vi "Async Read&Write.vi"(1 "Minor Frame Freq":u16 caption="Minor Frame Time", 4 "Frame Info Array":T1[](array[typedef]), 5 "Port":string, 6 "Stop Notification":refnum<notifier>, 7 "Main Engine Response Q":refnum<queue>, 8 "error in":errorcluster, 9 "Interupt Q":refnum<queue>, 10 "TCP Engine Response Q":refnum<queue>, 11 "Data Cluster":T3={"Array"=[], "Boolean"=FALSE, "Varient Data"=variant(string ""), "Stop Notification"=refnum, "Start Notification"=refnum, "Command Q"=refnum, "Main Engine Response Q"=refnum, "TCP Engine Response Q"=refnum, "Engine Name"="", "Log File Refnum"=refnum, "Async serial Configuration Cluster"={"Port"="", "Minor Frame Freq"=0, "Minor Frame Count"=0, "Frame Info"=[], "Sensor Type"=0, "OIM Address"=0}, "VISA resource name"="", "Y"=[], "Rate"=0, "Dynamic Data?"=FALSE, "DyData Not Received"=FALSE, "Interupt Q"=refnum, "Modbus"=refnum} {"Async serial Configuration Cluster"."Minor Frame Count" min=5 max=8 step=1}) -> (0 "error out":errorcluster, 2 "Total # Send":i32, 3 "Device Stop":bool)   [LabVIEW 2024]
doc: "All Rights Reserved © 2017 SyncSols"
uses:
  TCP Engine/Controls/TCP Engine Serial Interupt Cluster.ctl
  Controls/Async Frame Info Cluster.ctl
  Controls/Async Message Info Cluster.ctl
  Controls/Async Serial State Machine Data Cluster.ctl
  <vilib>/Modbus/master/Modbus Master.lvclass
  Controls/Async Serial Command Q Cluster.ctl
  Controls/Async Serial Configuration Cluster.ctl
  Main Engine/Controls/Main Engine JSON Command State.ctl
  Controls/Async Sensor Type.ctl
  <vilib>/Platform/TimedLoop/XDataNode/timing_clust.ctl
  <vilib>/Platform/TimedLoop/XDataNode/nitl_modes.ctl
  <vilib>/Platform/TimedLoop/XDataNode/wakeup.ctl
  1c283609-df89-4253-93f7-a40e07c9ee0e.vi
  <vilib>/Platform/TimedLoop/XDataNode/XDataNode.xnode
  <vilib>/Platform/TimedLoop/XDataNode/XDNodeRunTimeDep.lvlib
  TCP Engine/TCP Engine.lvlib
panel:
  in  "Frame Info":T1[](array[typedef])=[{"Frame ID"=1, "Message Info"=[{"Message"=[0, 0, 0, 0, 0, 0], "Message Name"="Camera cmd 1"}, {"Message"=[0, 0, 0, 0, 0, 0], "Message Name"="Camera cmd 2"}]}]
  out "Stop":bool=TRUE
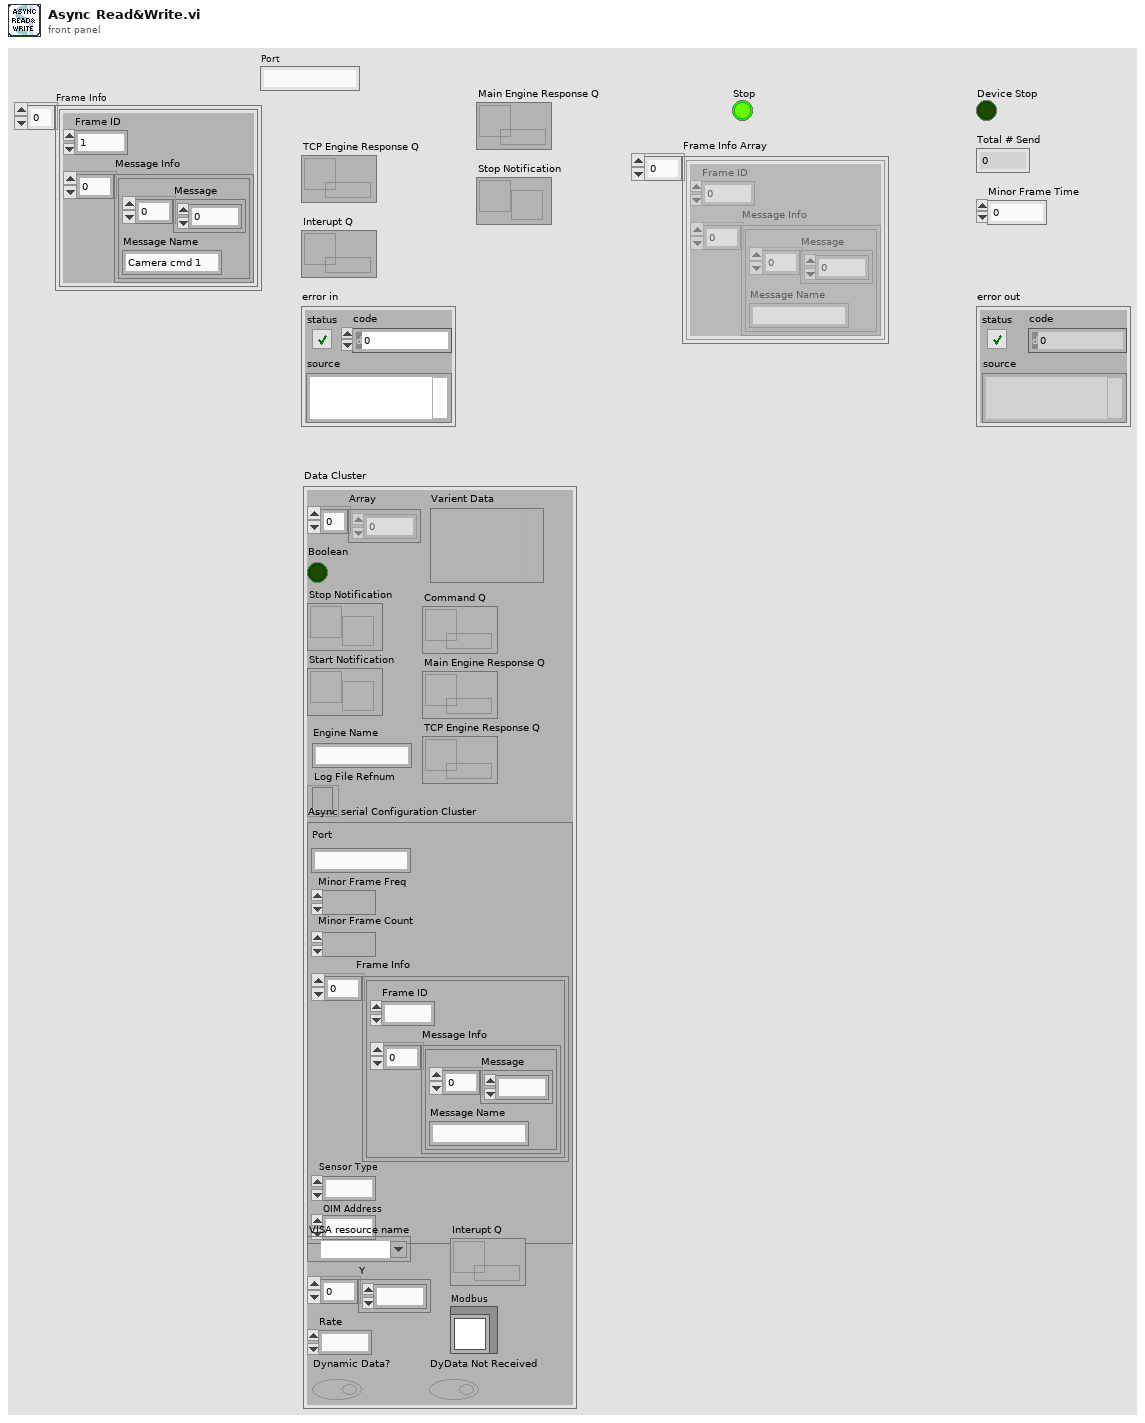
[diagram p1: front panel]
types:
  T1 = typedef "Async Frame Info Cluster.ctl" = cluster{"Frame ID":u16, "Message Info":T2[]}
  T2 = typedef "Async Message Info Cluster.ctl" = cluster{"Message":u8[], "Message Name":string}
  T3 = typedef "Async Serial State Machine Data Cluster.ctl" = cluster{"Array":dbl[], "Boolean":bool, "Varient Data":variant, "Stop Notification":refnum<notifier>, "Start Notification":refnum<notifier>, "Command Q":refnum<queue>, "Main Engine Response Q":refnum<queue>, "TCP Engine Response Q":refnum<queue>, "Engine Name":string, "Log File Refnum":refnum<file>, "Async serial Configuration Cluster":T4, "VISA resource name":refnum<visa-resource-name>, "Y":dbl[], "Rate":i32, "Dynamic Data?":bool, "DyData Not Received":bool, "Interupt Q":refnum<queue>, "Modbus":refnum<class "Modbus Master.lvclass">}
  T4 = typedef "Async Serial Configuration Cluster.ctl" = cluster{"Port":string, "Minor Frame Freq":u16, "Minor Frame Count":u16, "Frame Info":T1[], "Sensor Type":u16, "OIM Address":u16}
  T5 = typedef "Async Sensor Type.ctl" = enum16{"Camera", "INS", "Pri BMS", "Aux BMS", "Depth Sensor", "Altimeter", "OIM", "Thruster", "Acoustic Modem", "LED"}
  T6 = cluster{"Command":string, "SubCmd":string, "Data":cluster{"Port":string, "Length":u16, "Data":u8[], "Time":string}}
  T7 = typedef "XDNodeRunTimeDep.lvlib/timing_clust.ctl" = cluster{"Expected End [f-1]":u64, "Actual End [f-1]":u64, "Finished Late? [f-1]":bool, "Expected End [i-1]":u64, "Actual End [i-1]":u64, "Finished Late? [i-1]":bool, "Expected Start [i]":u64, "Actual Start [i]":u64, "Expected Start [f]":u64, "Actual Start [f]":u64, "Source Name":string, "Structure Name":string, "Period":i64, "Deadline":i64, "Offset":i64, "Start":i64, "Priority":i32, "Timeout":i32, "Mode":T8, "Wakeup Reason":T9, "Error":errorcluster, "Source Type":string, "Secondary Source Type":string, "Global End Time":u64, "Global Start Time":u64, "Frame Duration":u64, "Iteration Duration":u64, "Assigned CPU":i32, "I/O Scan Engine Mode":u32}
  T8 = typedef "XDNodeRunTimeDep.lvlib/nitl_modes.ctl" = enum32{"No Change", "Process missed periods, maintain original phase", "Discard missed periods, maintain original phase", "Process missed periods, ignore original phase", "Discard missed periods, ignore original phase"}
  T9 = typedef "XDNodeRunTimeDep.lvlib/wakeup.ctl" = enum32{"Normal", "Aborted", "Asynchronous wakeup", "Timing source error", "Timed loop error", "Timeout"}
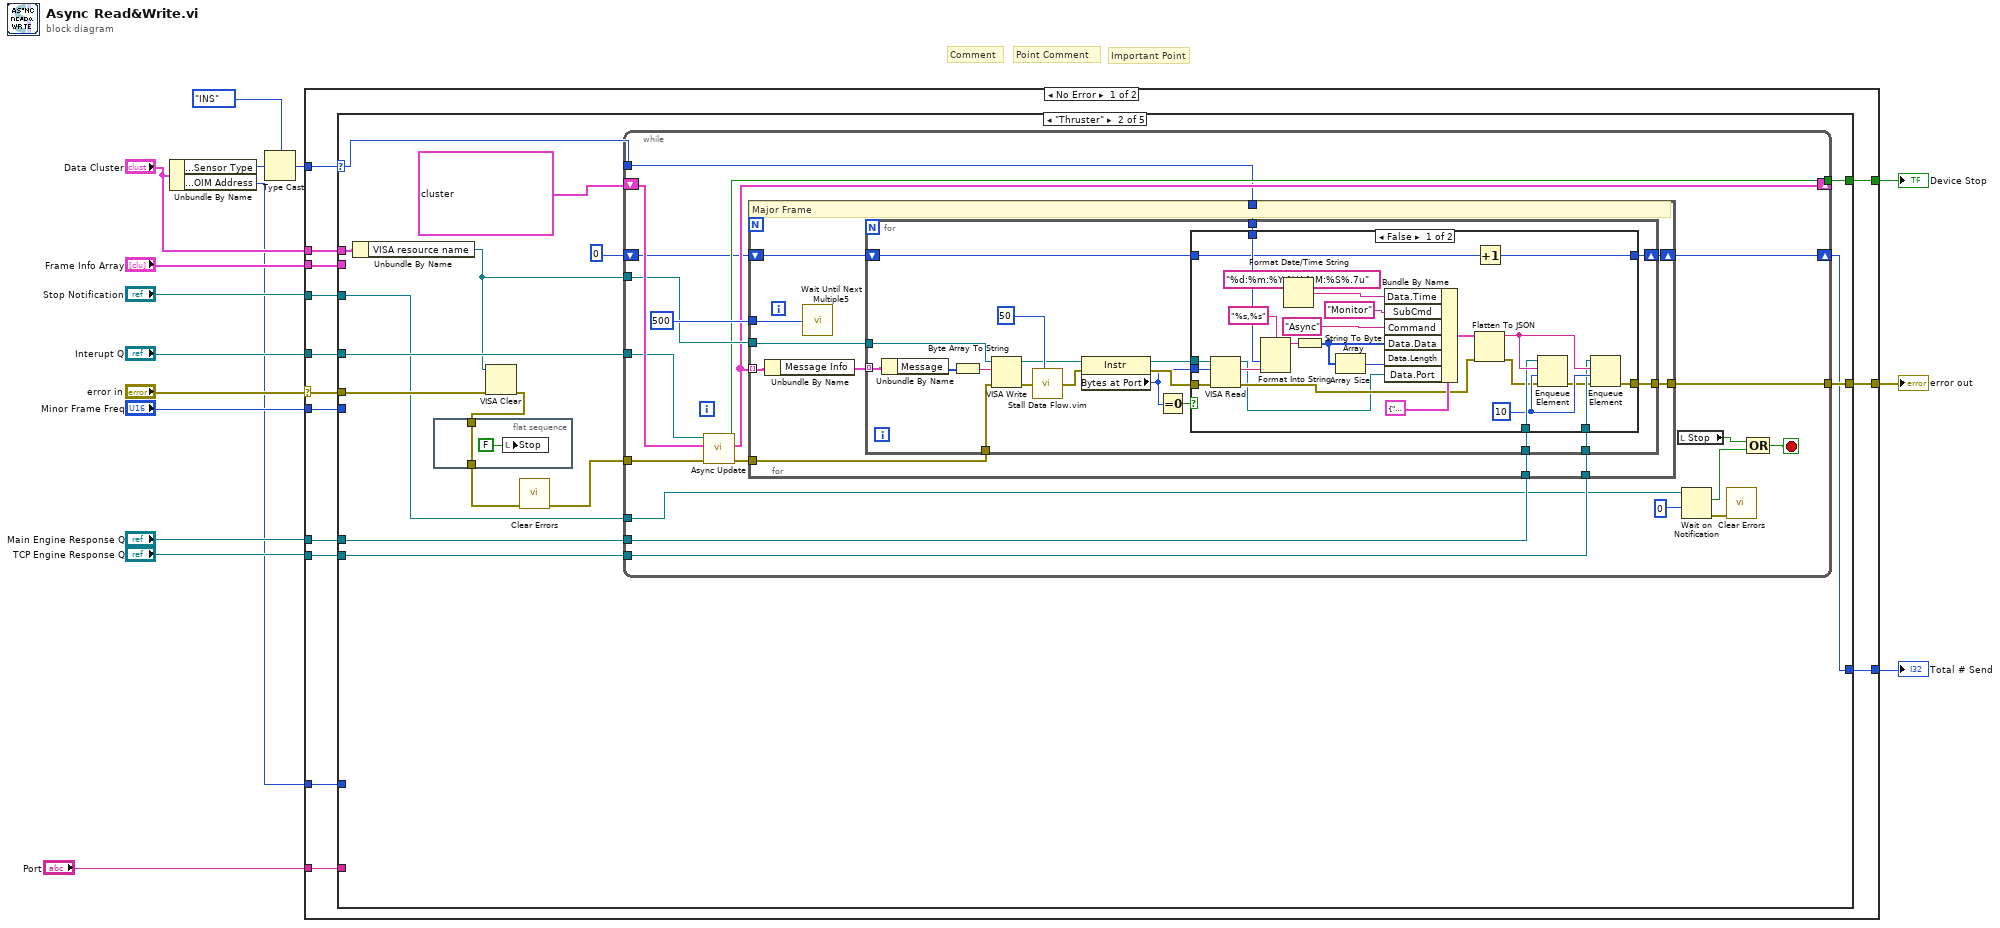
[diagram p0: block diagram]
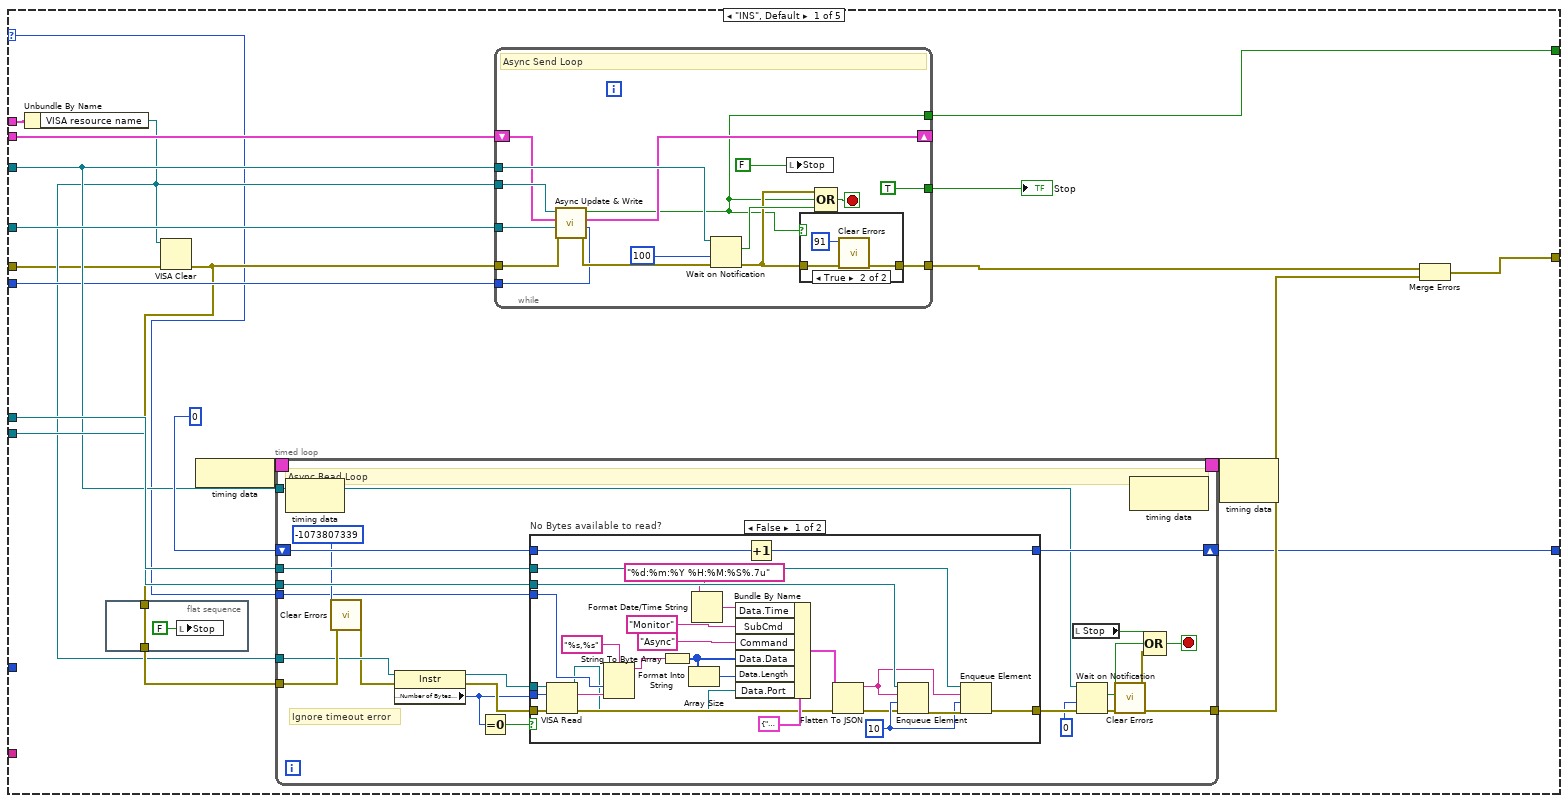
[diagram p2: hidden frame]
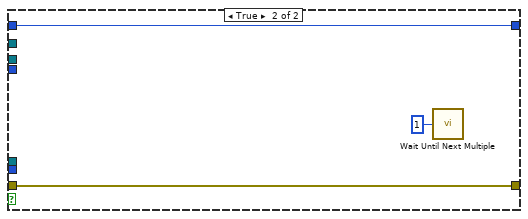
[diagram p3: hidden frame]
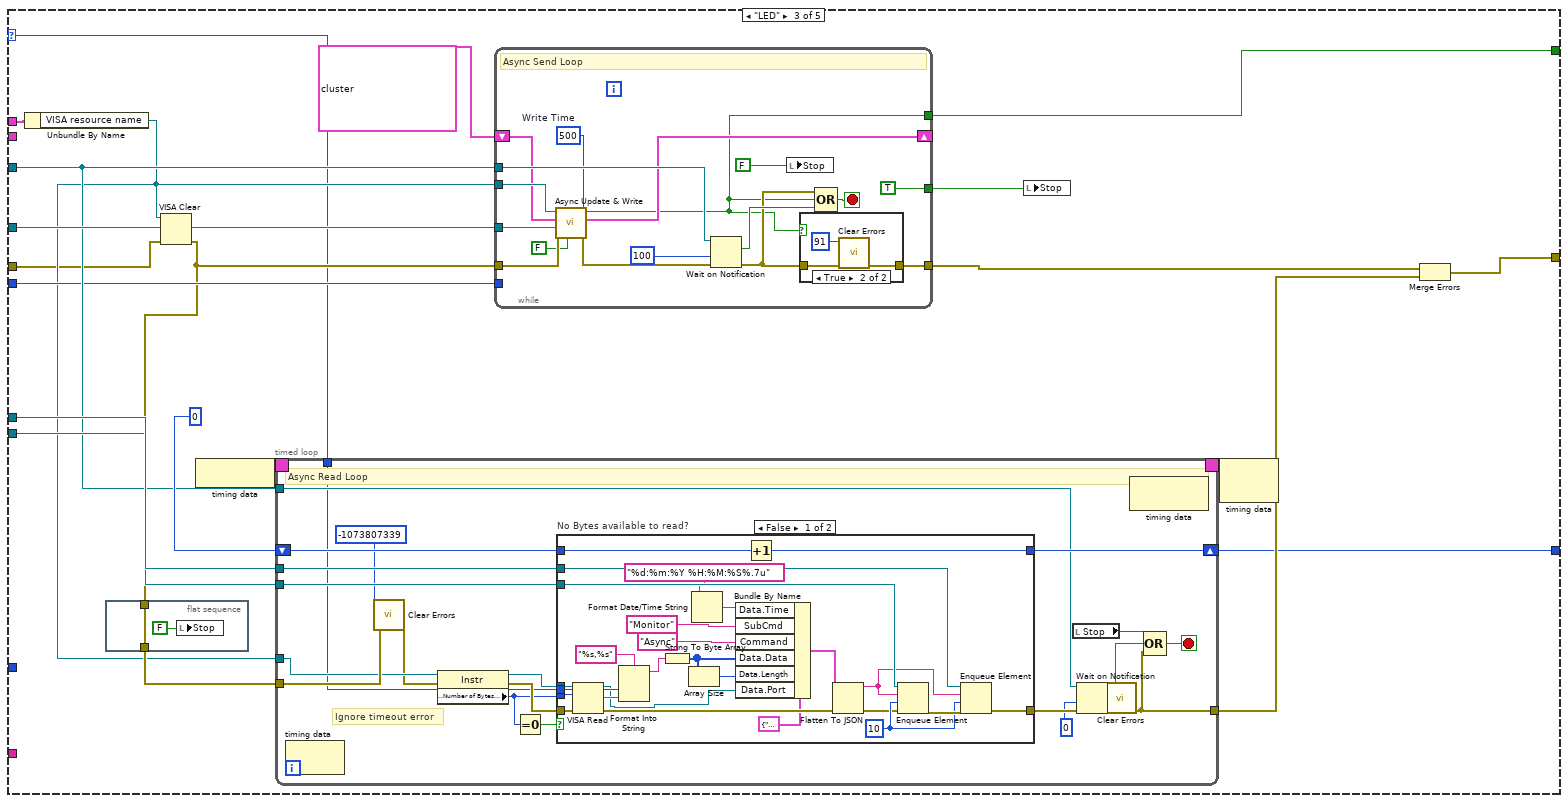
[diagram p6: hidden frame]
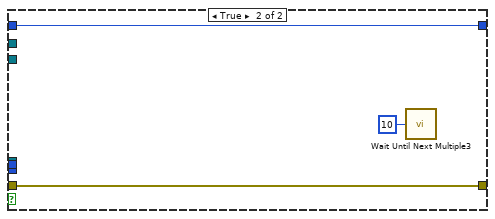
[diagram p7: hidden frame]
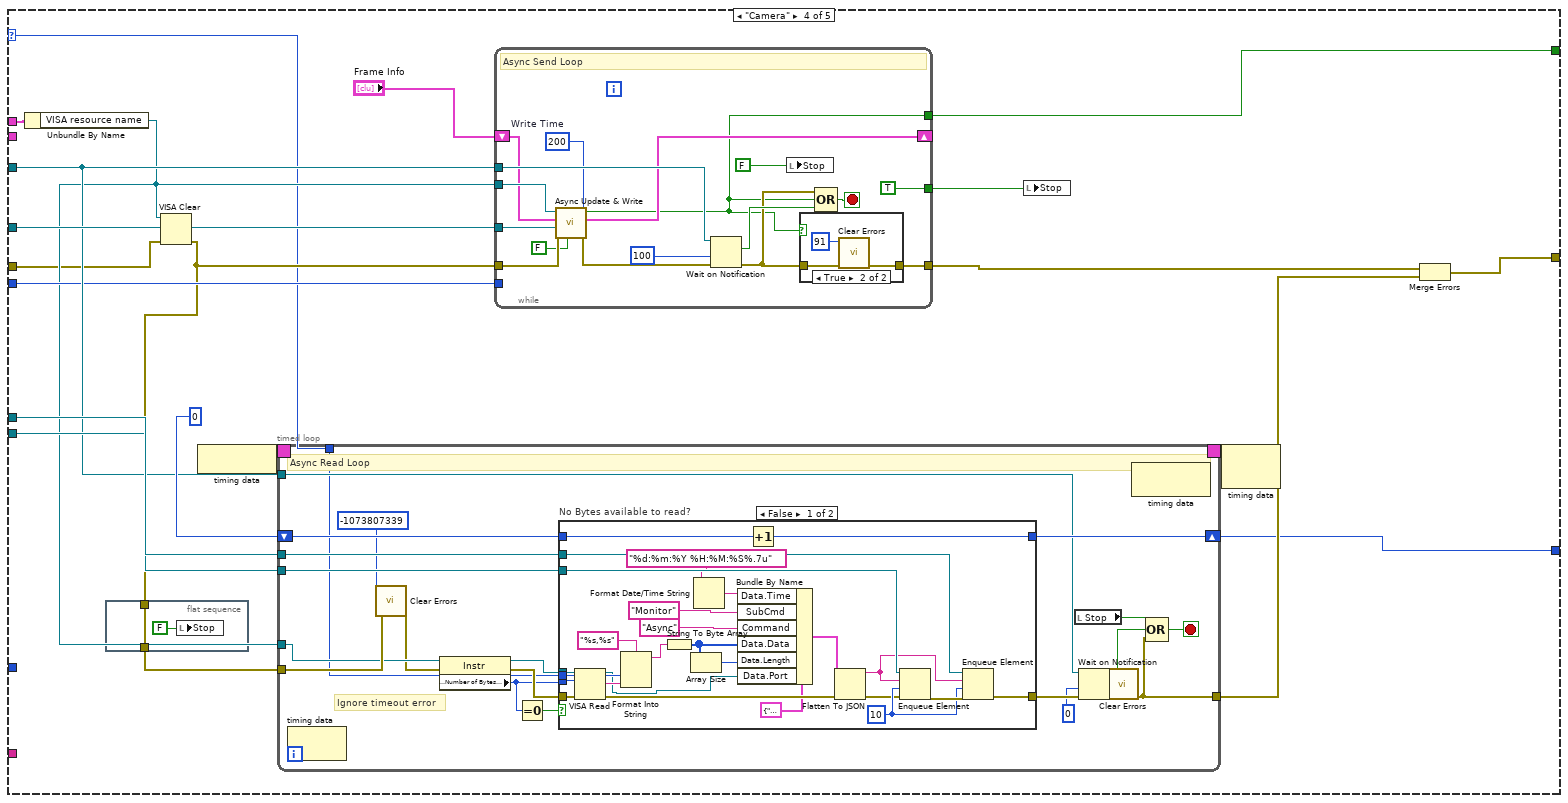
[diagram p9: hidden frame]
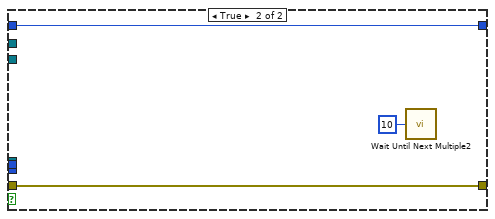
[diagram p10: hidden frame]
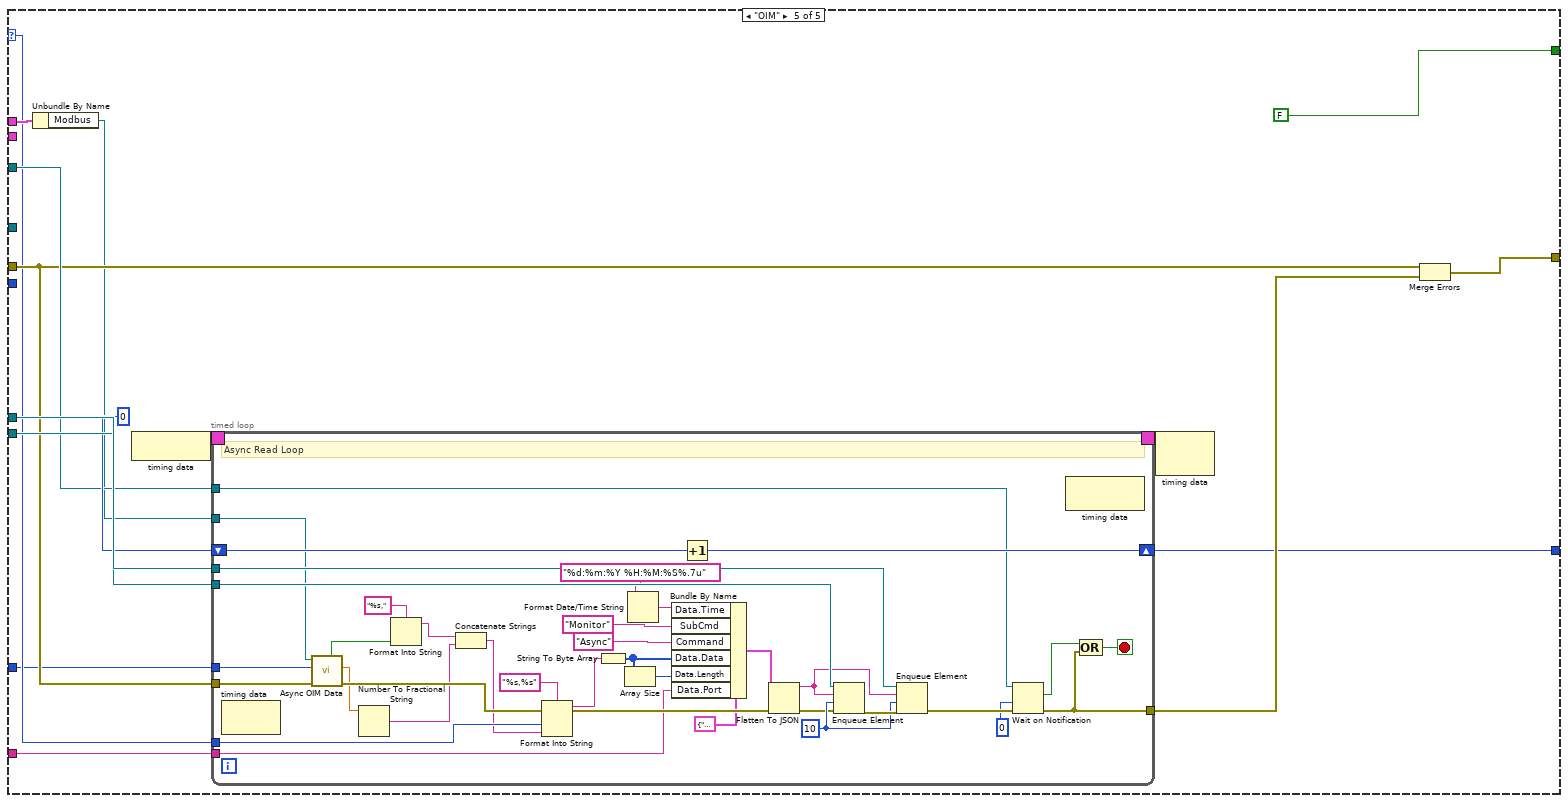
[diagram p12: hidden frame]
diagram:
  # "Important Point"
  # "Point Comment"
  # "Comment"
  n1 = Unbundle By Name("Data Cluster") -> ("Async serial Configuration Cluster.Sensor Type"=w7:u16, "Async serial Configuration Cluster.OIM Address"=w1:u16)
  n2 = Type Cast(type=Async_Sensor_Type."INS" ("Sensor Type"), x=w7) -> (*(type *) &x=w6:T5)
  n3 = case shown="No Error" "error in" {
    selector: "error in" -> [w21 w476]
    tunnel: [w23 w476] -> w16
    tunnel: "Stop Notification" -> [w26 _]
    tunnel: "Interupt Q" -> [w30 _]
    tunnel: "Main Engine Response Q" -> [w29 _]
    tunnel: "TCP Engine Response Q" -> [w28 _]
    tunnel: [w27 _] -> w2
    tunnel: "Frame Info Array" -> [w22 _]
    tunnel: "Minor Frame Freq" -> [w25 _]
    tunnel: [w24 _] -> w9
    tunnel: w6 -> [w20 _]
    tunnel: "Data Cluster" -> [w19 _]
    tunnel: "Port" -> [w18 _]
    tunnel: w1 -> [w17 _]
    frame No Error {
      n4 = case shown="\"Thruster\"" w20 {
        selector: w20 -> [w32 w137 w227 w325 w423]
        tunnel: w30 -> [w48 w141 w241 w339 _]
        tunnel: w29 -> [w47 w133 w240 w338 w433]
        tunnel: w28 -> [w46 w132 w239 w337 w432]
        tunnel: [w31 w128 w224 w322 w421] -> w27
        tunnel: w26 -> [w44 w130 w237 w335 w430]
        tunnel: w25 -> [w43 _ w236 w334 _]
        tunnel: [w42 w138 w235 w333 FALSE ("Stop")] -> w24
        tunnel: [w41 w129 w234 w332 w429] -> w23
        tunnel: w22 -> [w37 _ _ _ _]
        tunnel: w21 -> [w34 w142 w229 w327 w427]
        tunnel: w19 -> [w36 w143 w231 w329 w425]
        tunnel: w18 -> [_ _ _ _ w422]
        tunnel: w17 -> [_ _ _ _ w420]
        frame "INS", Default {
          n5 = Unbundle By Name(w36) -> ("VISA resource name"=w35:refnum<visa-resource-name>)
          n6 = flat-sequence {
            tunnel: w33 -> [w106]
            tunnel: [w106] -> w38
            frame #0 {
              n7 = local write "Stop"(FALSE ("Recive Stop")) -> ()
            }
          }
          n8 = VISA Clear(VISA resource name=w35, error in (no error)=w34) -> (error out=w33:errorcluster)  [unwired: 1 out]
          n9 = node-c288() -> (w51:T7)
          n10 = timed-loop {
            tunnel: w38 -> [w61]
            tunnel: w47 -> [w72]
            tunnel: w46 -> [w71]
            shift-right: [w69] -> w31
            shift-left: 0 -> [w70]
            tunnel: w44 -> [w67]
            tunnel: [w52] -> w40
            tunnel: w35 -> [w60]
            timing: w51 -> [_]
            timing-out: [_] -> w50
            tunnel: w32 -> [w53]
            stop <- w64 stop-if-true
            # "Ignore timeout error"
            # "Async Read Loop"
            n11 = node-c288() -> ()  [unwired: 1 in, 1 out]
            n12 = call <vilib>:"Clear Errors.vi"("error in (no error)"=w61, "specific error code to clear (0: all)"=-1073807339) -> ("error out"=w58:errorcluster)  [unwired: 4 in, 1 out]
            n13 = property class="Instr"(reference=w60, error in=w58) -> (reference out=w57:refnum<visa-resource-name>, error out=w56:errorcluster, "Serial Settings:Number of Bytes at Serial Port"=w55:u32)
            n14 = Equal To 0?(x=w55) -> (x = 0?=w54:bool)
            n15 = case "No Bytes available to read?" shown="False" w54 {
              tunnel: w72 -> [w93 _]
              tunnel: w71 -> [w98 _]
              tunnel: w57 -> [w77 _]
              tunnel: w55 -> [w74 _]
              tunnel: w56 -> [w78 w100]
              tunnel: w70 -> [w88 w101]
              tunnel: [w87 w101] -> w69
              tunnel: [w86 w100] -> w68
              tunnel: w53 -> [w80 _]
              frame False {
                w96 = 10 ("timeout in ms (-1)")
                n16 = VISA Read(VISA resource name=w77, byte count=w74, error in (no error)=w78) -> (VISA resource name out=w73:refnum<visa-resource-name>, read buffer=w76:string, error out=w75:errorcluster)  [unwired: 1 out]
                n17 = Format Into String(format string="%s,%s", w80, w76) -> (resulting string=w81:string)  [unwired: 2 in, 1 out]
                n18 = String To Byte Array(string=w81) -> (unsigned byte array=w90:u8[])
                n19 = Array Size(array=w90) -> (size(s)=w89:i32)
                n20 = Format Date/Time String(time format string (%c)="%d:%m:%Y %H:%M:%S%.7u") -> (date/time string=w84:string)  [unwired: 2 in]
                n21 = Bundle By Name(cluster=T6 {"Command"="", "SubCmd"="", "Data"={"Port"="", "Length"=0, "Data"=[], "Time"=""}}, "Data.Time"=w84, "SubCmd"="Monitor" ("Sub Command"), "Command"="Async", "Data.Data"=w90, "Data.Length"=w89, "Data.Port"=w73) -> (w79:T6)
                n22 = Increment(x=w88) -> (x+1=w87:i32)
                n23 = Flatten To JSON(anything=w79, error in (no error)=w75) -> (JSON string=w95:string, 11:w94:errorcluster)  [unwired: 1 in]
                n24 = Enqueue Element(queue=w98, element=w95, timeout in ms (-1)=w96, error in (no error)=w94) -> (error out=w97:errorcluster)  [unwired: 2 out]
                n25 = Enqueue Element(queue=w93, element=w95, timeout in ms (-1)=w96, error in (no error)=w97) -> (error out=w86:errorcluster)  [unwired: 2 out]
              }
              frame True {
                n26 = call "Wait Until Next Multiple"("Count(uSec)"=u32 1) -> ()  [unwired: 1 out]
              }
            }
            n27 = local read "Stop"() -> (w62:bool)
            n28 = Wait on Notification(notifier=w67, timeout in ms (-1)=0, error in (no error)=w68) -> (notification=w65:bool, error out=w63:errorcluster)  [unwired: 1 in, 2 out]
            n29 = call <vilib>:"Clear Errors.vi"("error in (no error)"=w63) -> ("error out"=w52:errorcluster)  [unwired: 5 in, 1 out]
            n30 = node-c288() -> ()  [unwired: 1 in, 1 out]
            n31 = Compound Arithmetic op=OR(w62, w65, w52) -> (w64:bool)
          }
          n32 = while {
            tunnel: w48 -> [w117]
            tunnel: w44 -> [w120]
            tunnel: [w119] -> w49
            tunnel: w33 -> [w111]
            tunnel: w35 -> [w118]
            shift-right: [w116] -> _
            shift-left: w37 -> [w110]
            tunnel: w43 -> [w109]
            tunnel: [w114] -> w42
            tunnel: [TRUE] -> w39
            stop <- w123 stop-if-true
            # "Async Send Loop"
            n33 = call "Async Update & Write.vi"("Minor Frame Freq"=w109, "error in"=w111, "Interupt Q"=w117, "Frame Info Array"=w110, "Visa"=w118) -> ("error out"=w115:errorcluster, "Frame Info Array"=w116:T1[], "Stop"=w114:bool)  [unwired: 4 in]
            n34 = Wait on Notification(notifier=w120, timeout in ms (-1)=100 ("t"), error in (no error)=w115) -> (notification=w122:bool, error out=w121:errorcluster)  [unwired: 1 in, 2 out]
            n35 = local write "Stop"(FALSE) -> ()
            n36 = case shown="True" w114 {
              tunnel: w121 -> [w124 w127]
              tunnel: [w124 w126] -> w119
              frame False {
              }
              frame True {
                n37 = call <vilib>:"Clear Errors.vi"("error in (no error)"=w127, "specific error code to clear (0: all)"=91) -> ("error out"=w126:errorcluster)  [unwired: 4 in, 1 out]
              }
            }
            n38 = Compound Arithmetic op=OR(w121, w114, w122) -> (w123:bool)
          }
          "Stop" <- w39
          n39 = node-c288(w50) -> ()  [unwired: 1 out]
          n40 = Merge Errors(w49, w40) -> (w41:errorcluster)
        }
        frame "Thruster" {
          n41 = Unbundle By Name(w143) -> ("VISA resource name"=w140:refnum<visa-resource-name>)
          n42 = flat-sequence {
            tunnel: w136 -> [w222]
            tunnel: [w222] -> w135
            frame #0 {
              n43 = local write "Stop"(FALSE ("Recive Stop")) -> ()
            }
          }
          n44 = VISA Clear(VISA resource name=w140, error in (no error)=w142) -> (error out=w136:errorcluster)  [unwired: 1 out]
          n45 = call <vilib>:"Clear Errors.vi"("error in (no error)"=w135) -> ("error out"=w134:errorcluster)  [unwired: 5 in, 1 out]
          n46 = while {
            tunnel: w141 -> [w161]
            tunnel: w140 -> [w159]
            shift-right: [w158] -> _
            shift-left: T1[] [{"Frame ID"=1, "Message Info"=[{"Message"=[16, 1, 111, 50, 0, 0, 0, 0, 16, 3, 197], "Message Name"="Astatus"}]}, {"Frame ID"=2, "Message Info"=[{"Message"=[16, 1, 111, 65, 32, 32, 0, 0, 16, 3, 20], "Message Name"="cmd"}]}, {"Frame ID"=3, "Message Info"=[{"Message"=[16, 1, 111, 55, 0, 0, 0, 0, 16, 3, 202], "Message Name"="Drstatus"}]}] ("Frame Info 2") -> [w162]
            tunnel: w134 -> [w160]
            tunnel: [w144] -> w129
            tunnel: [w157] -> w138
            tunnel: w137 -> [w156]
            tunnel: w133 -> [w155]
            tunnel: w132 -> [w154]
            shift-right: [w151] -> w128
            shift-left: 0 -> [w152]
            tunnel: w130 -> [w146]
            stop <- w145 stop-if-true
            n47 = call "Async Update.vi"("error in"=w160, "Frame Info Array"=w162, "Interupt Q"=w161) -> ("error out"=w153:errorcluster, "Frame Info Array"=w158:T1[], "Stop"=w157:bool)  [unwired: 5 in, 1 out]
            n48 = for {
              tunnel: w159 -> [w172]
              tunnel: u16 500 ("Minor Frame Freq 2") -> [w173]
              tunnel: w158 -> [w170] mode=indexing
              tunnel: w153 -> [w171]
              tunnel: w156 -> [w169]
              tunnel: w155 -> [w168]
              tunnel: w154 -> [w167]
              shift-right: [w165] -> w151
              shift-left: w152 -> [w166]
              tunnel: [w164] -> w144
              # "Major Frame"
              n49 = Unbundle By Name(w170) -> ("Message Info"=w174:T2[])
              n50 = call "Wait Until Next Multiple5"("Count(mSec)"=w173) -> ()  [unwired: 1 out]
              n51 = for {
                tunnel: w174 -> [w193] mode=indexing
                tunnel: w172 -> [w190]
                tunnel: w171 -> [w189]
                tunnel: w169 -> [w182]
                tunnel: w168 -> [w181]
                tunnel: w167 -> [w180]
                shift-right: [w176] -> w165
                shift-left: w166 -> [w177]
                tunnel: [w175] -> w164
                n52 = Unbundle By Name(w193) -> ("Message"=w192:u8[])
                n53 = Byte Array To String(unsigned byte array=w192) -> (string=w191:string)
                n54 = VISA Write(VISA resource name=w190, write buffer=w191, error in (no error)=w189) -> (VISA resource name out=w186:refnum<visa-resource-name>, error out=w188:errorcluster)  [unwired: 1 out]
                n55 = call "Stall Data Flow.vim"("value in"=w188, "milliseconds to wait"=u32 50) -> ("value out"=w185:errorcluster)  [unwired: 1 out]
                n56 = property class="Instr"(reference=w186, error in=w185) -> (reference out=w183:refnum<visa-resource-name>, error out=w184:errorcluster, "Bytes at Port"=w179:u32)
                n57 = Equal To 0?(x=w179) -> (x = 0?=w178:bool)
                n58 = case shown="False" w178 {
                  tunnel: w184 -> [w219 w220]
                  tunnel: w179 -> [w218 _]
                  tunnel: w183 -> [w217 _]
                  tunnel: w182 -> [w215 _]
                  tunnel: w181 -> [w203 _]
                  tunnel: w180 -> [w200 _]
                  tunnel: w177 -> [w198 w221]
                  tunnel: [w197 w221] -> w176
                  tunnel: [w196 w220] -> w175
                  frame False {
                    w202 = 10 ("timeout in ms (-1)")
                    n59 = VISA Read(VISA resource name=w217, byte count=w218, error in (no error)=w219) -> (VISA resource name out=w195:refnum<visa-resource-name>, read buffer=w214:string, error out=w205:errorcluster)  [unwired: 1 out]
                    n60 = Format Into String(format string="%s,%s", w215, w214) -> (resulting string=w208:string)  [unwired: 2 in, 1 out]
                    n61 = Format Date/Time String(time format string (%c)="%d:%m:%Y %H:%M:%S%.7u") -> (date/time string=w211:string)  [unwired: 2 in]
                    n62 = String To Byte Array(string=w208) -> (unsigned byte array=w206:u8[])
                    n63 = Array Size(array=w206) -> (size(s)=w207:i32)
                    n64 = Bundle By Name(cluster=T6 {"Command"="", "SubCmd"="", "Data"={"Port"="", "Length"=0, "Data"=[], "Time"=""}}, "Data.Time"=w211, "SubCmd"="Monitor", "Command"="Async" ("SubCmd"), "Data.Data"=w206, "Data.Length"=w207, "Data.Port"=w195) -> (w194:T6)
                    n65 = Flatten To JSON(anything=w194, error in (no error)=w205) -> (JSON string=w204:string, 11:w201:errorcluster)  [unwired: 1 in]
                    n66 = Increment(x=w198) -> (x+1=w197:i32)
                    n67 = Enqueue Element(queue=w203, element=w204, timeout in ms (-1)=w202, error in (no error)=w201) -> (error out=w199:errorcluster)  [unwired: 2 out]
                    n68 = Enqueue Element(queue=w200, element=w204, timeout in ms (-1)=w202, error in (no error)=w199) -> (error out=w196:errorcluster)  [unwired: 2 out]
                  }
                  frame True {
                  }
                }
              }
            }
            n69 = local read "Stop"() -> (w150:bool)
            n70 = Wait on Notification(notifier=w146, timeout in ms (-1)=0) -> (notification=w148:bool, error out=w149:errorcluster)  [unwired: 2 in, 2 out]
            n71 = call <vilib>:"Clear Errors.vi"("error in (no error)"=w149) -> ()  [unwired: 5 in, 2 out]
            n72 = Compound Arithmetic op=OR(w150, w148) -> (w145:bool)
          }
        }
        frame "LED" {
          n73 = Unbundle By Name(w231) -> ("VISA resource name"=w230:refnum<visa-resource-name>)
          n74 = flat-sequence {
            tunnel: w228 -> [w299]
            tunnel: [w299] -> w232
            frame #0 {
              n75 = local write "Stop"(FALSE ("Recive Stop")) -> ()
            }
          }
          n76 = VISA Clear(VISA resource name=w230, error in (no error)=w229) -> (error out=w228:errorcluster)  [unwired: 1 out]
          n77 = node-c288() -> (w244:T7)
          n78 = timed-loop {
            tunnel: w232 -> [w254]
            tunnel: w240 -> [w265]
            tunnel: w239 -> [w264]
            shift-right: [w262] -> w224
            shift-left: 0 -> [w263]
            tunnel: w237 -> [w260]
            tunnel: [w245] -> w233
            tunnel: w230 -> [w253]
            timing: w244 -> [_]
            timing-out: [_] -> w243
            tunnel: w227 -> [w246]
            stop <- w257 stop-if-true
            # "Ignore timeout error"
            # "Async Read Loop"
            n79 = node-c288() -> ()  [unwired: 1 in, 1 out]
            n80 = call <vilib>:"Clear Errors.vi"("error in (no error)"=w254, "specific error code to clear (0: all)"=-1073807339) -> ("error out"=w251:errorcluster)  [unwired: 4 in, 1 out]
            n81 = property class="Instr"(reference=w253, error in=w251) -> (reference out=w250:refnum<visa-resource-name>, error out=w249:errorcluster, "Serial Settings:Number of Bytes at Serial Port"=w248:u32)
            n82 = Equal To 0?(x=w248) -> (x = 0?=w247:bool)
            n83 = case "No Bytes available to read?" shown="False" w247 {
              tunnel: w265 -> [w282 _]
              tunnel: w264 -> [w291 _]
              tunnel: w250 -> [w285 _]
              tunnel: w248 -> [w284 _]
              tunnel: w249 -> [w283 w293]
              tunnel: w263 -> [w276 w294]
              tunnel: [w275 w294] -> w262
              tunnel: [w274 w293] -> w261
              tunnel: w246 -> [w267 _]
              frame False {
                w289 = 10 ("timeout in ms (-1)")
                n84 = VISA Read(VISA resource name=w285, byte count=w284, error in (no error)=w283) -> (VISA resource name out=w266:refnum<visa-resource-name>, read buffer=w269:string, error out=w287:errorcluster)  [unwired: 1 out]
                n85 = Format Into String(format string="%s,%s", w267, w269) -> (resulting string=w268:string)  [unwired: 2 in, 1 out]
                n86 = String To Byte Array(string=w268) -> (unsigned byte array=w278:u8[])
                n87 = Array Size(array=w278) -> (size(s)=w277:i32)
                n88 = Format Date/Time String(time format string (%c)="%d:%m:%Y %H:%M:%S%.7u") -> (date/time string=w272:string)  [unwired: 2 in]
                n89 = Bundle By Name(cluster=T6 {"Command"="", "SubCmd"="", "Data"={"Port"="", "Length"=0, "Data"=[], "Time"=""}}, "Data.Time"=w272, "SubCmd"="Monitor" ("Sub Command"), "Command"="Async", "Data.Data"=w278, "Data.Length"=w277, "Data.Port"=w266) -> (w281:T6)
                n90 = Increment(x=w276) -> (x+1=w275:i32)
                n91 = Flatten To JSON(anything=w281, error in (no error)=w287) -> (JSON string=w288:string, 11:w286:errorcluster)  [unwired: 1 in]
                n92 = Enqueue Element(queue=w291, element=w288, timeout in ms (-1)=w289, error in (no error)=w286) -> (error out=w290:errorcluster)  [unwired: 2 out]
                n93 = Enqueue Element(queue=w282, element=w288, timeout in ms (-1)=w289, error in (no error)=w290) -> (error out=w274:errorcluster)  [unwired: 2 out]
              }
              frame True {
                n94 = call "Wait Until Next Multiple3"("Count(uSec)"=u32 10) -> ()  [unwired: 1 out]
              }
            }
            n95 = local read "Stop"() -> (w255:bool)
            n96 = Wait on Notification(notifier=w260, timeout in ms (-1)=0, error in (no error)=w261) -> (notification=w258:bool, error out=w256:errorcluster)  [unwired: 1 in, 2 out]
            n97 = call <vilib>:"Clear Errors.vi"("error in (no error)"=w256) -> ("error out"=w245:errorcluster)  [unwired: 5 in, 1 out]
            n98 = node-c288() -> ()  [unwired: 1 in, 1 out]
            n99 = Compound Arithmetic op=OR(w255, w258, w245) -> (w257:bool)
          }
          n100 = while {
            tunnel: w241 -> [w311]
            tunnel: w237 -> [w314]
            tunnel: [w313] -> w242
            tunnel: w228 -> [w305]
            tunnel: w230 -> [w312]
            shift-right: [w310] -> _
            shift-left: T1[] [{"Frame ID"=1, "Message Info"=[{"Message"=[0], "Message Name"="LED"}]}] ("Frame Info") -> [w304]
            tunnel: w236 -> [_]
            tunnel: [w308] -> w235
            tunnel: [TRUE] -> w225
            stop <- w317 stop-if-true
            w302 = u16 500  # Write Time
            # "Async Send Loop"
            n101 = call "Async Update & Write.vi"("Minor Frame Freq"=w302, "Continuous Tx"=FALSE, "error in"=w305, "Interupt Q"=w311, "Frame Info Array"=w304, "Visa"=w312) -> ("error out"=w309:errorcluster, "Frame Info Array"=w310:T1[], "Stop"=w308:bool)  [unwired: 3 in]
            n102 = Wait on Notification(notifier=w314, timeout in ms (-1)=100 ("t"), error in (no error)=w309) -> (notification=w316:bool, error out=w315:errorcluster)  [unwired: 1 in, 2 out]
            n103 = local write "Stop"(FALSE) -> ()
            n104 = case shown="True" w308 {
              tunnel: w315 -> [w318 w321]
              tunnel: [w318 w320] -> w313
              frame False {
              }
              frame True {
                n105 = call <vilib>:"Clear Errors.vi"("error in (no error)"=w321, "specific error code to clear (0: all)"=91) -> ("error out"=w320:errorcluster)  [unwired: 4 in, 1 out]
              }
            }
            n106 = Compound Arithmetic op=OR(w315, w308, w316) -> (w317:bool)
          }
          n107 = local write "Stop"(w225) -> ()
          n108 = node-c288(w243) -> ()  [unwired: 1 out]
          n109 = Merge Errors(w242, w233) -> (w234:errorcluster)
        }
        frame "Camera" {
          n110 = Unbundle By Name(w329) -> ("VISA resource name"=w328:refnum<visa-resource-name>)
          n111 = flat-sequence {
            tunnel: w326 -> [w397]
            tunnel: [w397] -> w330
            frame #0 {
              n112 = local write "Stop"(FALSE ("Recive Stop")) -> ()
            }
          }
          n113 = VISA Clear(VISA resource name=w328, error in (no error)=w327) -> (error out=w326:errorcluster)  [unwired: 1 out]
          n114 = node-c288() -> (w342:T7)
          n115 = timed-loop {
            tunnel: w330 -> [w352]
            tunnel: w338 -> [w363]
            tunnel: w337 -> [w362]
            shift-right: [w360] -> w322
            shift-left: 0 -> [w361]
            tunnel: w335 -> [w358]
            tunnel: [w343] -> w331
            tunnel: w328 -> [w351]
            timing: w342 -> [_]
            timing-out: [_] -> w341
            tunnel: w325 -> [w344]
            stop <- w355 stop-if-true
            # "Ignore timeout error"
            # "Async Read Loop"
            n116 = node-c288() -> ()  [unwired: 1 in, 1 out]
            n117 = call <vilib>:"Clear Errors.vi"("error in (no error)"=w352, "specific error code to clear (0: all)"=-1073807339) -> ("error out"=w349:errorcluster)  [unwired: 4 in, 1 out]
            n118 = property class="Instr"(reference=w351, error in=w349) -> (reference out=w348:refnum<visa-resource-name>, error out=w347:errorcluster, "Serial Settings:Number of Bytes at Serial Port"=w346:u32)
            n119 = Equal To 0?(x=w346) -> (x = 0?=w345:bool)
            n120 = case "No Bytes available to read?" shown="False" w345 {
              tunnel: w363 -> [w380 _]
              tunnel: w362 -> [w389 _]
              tunnel: w348 -> [w383 _]
              tunnel: w346 -> [w382 _]
              tunnel: w347 -> [w381 w391]
              tunnel: w361 -> [w374 w392]
              tunnel: [w373 w392] -> w360
              tunnel: [w372 w391] -> w359
              tunnel: w344 -> [w365 _]
              frame False {
                w387 = 10 ("timeout in ms (-1)")
                n121 = VISA Read(VISA resource name=w383, byte count=w382, error in (no error)=w381) -> (VISA resource name out=w364:refnum<visa-resource-name>, read buffer=w367:string, error out=w385:errorcluster)  [unwired: 1 out]
                n122 = Format Into String(format string="%s,%s", w365, w367) -> (resulting string=w366:string)  [unwired: 2 in, 1 out]
                n123 = String To Byte Array(string=w366) -> (unsigned byte array=w376:u8[])
                n124 = Array Size(array=w376) -> (size(s)=w375:i32)
                n125 = Format Date/Time String(time format string (%c)="%d:%m:%Y %H:%M:%S%.7u") -> (date/time string=w370:string)  [unwired: 2 in]
                n126 = Bundle By Name(cluster=T6 {"Command"="", "SubCmd"="", "Data"={"Port"="", "Length"=0, "Data"=[], "Time"=""}}, "Data.Time"=w370, "SubCmd"="Monitor" ("Sub Command"), "Command"="Async", "Data.Data"=w376, "Data.Length"=w375, "Data.Port"=w364) -> (w379:T6)
                n127 = Increment(x=w374) -> (x+1=w373:i32)
                n128 = Flatten To JSON(anything=w379, error in (no error)=w385) -> (JSON string=w386:string, 11:w384:errorcluster)  [unwired: 1 in]
                n129 = Enqueue Element(queue=w389, element=w386, timeout in ms (-1)=w387, error in (no error)=w384) -> (error out=w388:errorcluster)  [unwired: 2 out]
                n130 = Enqueue Element(queue=w380, element=w386, timeout in ms (-1)=w387, error in (no error)=w388) -> (error out=w372:errorcluster)  [unwired: 2 out]
              }
              frame True {
                n131 = call "Wait Until Next Multiple2"("Count(uSec)"=u32 10) -> ()  [unwired: 1 out]
              }
            }
            n132 = local read "Stop"() -> (w353:bool)
            n133 = Wait on Notification(notifier=w358, timeout in ms (-1)=0, error in (no error)=w359) -> (notification=w356:bool, error out=w354:errorcluster)  [unwired: 1 in, 2 out]
            n134 = call <vilib>:"Clear Errors.vi"("error in (no error)"=w354) -> ("error out"=w343:errorcluster)  [unwired: 5 in, 1 out]
            n135 = node-c288() -> ()  [unwired: 1 in, 1 out]
            n136 = Compound Arithmetic op=OR(w353, w356, w343) -> (w355:bool)
          }
          n137 = while {
            tunnel: w339 -> [w409]
            tunnel: w335 -> [w412]
            tunnel: [w411] -> w340
            tunnel: w326 -> [w403]
            tunnel: w328 -> [w410]
            shift-right: [w408] -> _
            shift-left: "Frame Info" -> [w402]
            tunnel: w334 -> [_]
            tunnel: [w406] -> w333
            tunnel: [TRUE] -> w323
            stop <- w415 stop-if-true
            w400 = u16 200  # Write Time
            # "Async Send Loop"
            n138 = call "Async Update & Write.vi"("Minor Frame Freq"=w400, "Continuous Tx"=FALSE, "error in"=w403, "Interupt Q"=w409, "Frame Info Array"=w402, "Visa"=w410) -> ("error out"=w407:errorcluster, "Frame Info Array"=w408:T1[], "Stop"=w406:bool)  [unwired: 3 in]
            n139 = Wait on Notification(notifier=w412, timeout in ms (-1)=100 ("t"), error in (no error)=w407) -> (notification=w414:bool, error out=w413:errorcluster)  [unwired: 1 in, 2 out]
            n140 = local write "Stop"(FALSE) -> ()
            n141 = case shown="True" w406 {
              tunnel: w413 -> [w416 w419]
              tunnel: [w416 w418] -> w411
              frame False {
              }
              frame True {
                n142 = call <vilib>:"Clear Errors.vi"("error in (no error)"=w419, "specific error code to clear (0: all)"=91) -> ("error out"=w418:errorcluster)  [unwired: 4 in, 1 out]
              }
            }
            n143 = Compound Arithmetic op=OR(w413, w406, w414) -> (w415:bool)
          }
          n144 = local write "Stop"(w323) -> ()
          n145 = node-c288(w341) -> ()  [unwired: 1 out]
          n146 = Merge Errors(w340, w331) -> (w332:errorcluster)
        }
        frame "OIM" {
          n147 = Unbundle By Name(w425) -> ("Modbus"=w424:refnum<class "Modbus Master.lvclass">)
          n148 = node-c288() -> (w435:T7)
          n149 = timed-loop {
            tunnel: w427 -> [w461]
            tunnel: w433 -> [w471]
            tunnel: w432 -> [w470]
            shift-right: [w468] -> w421
            shift-left: 0 -> [w469]
            tunnel: w430 -> [w466]
            tunnel: [w462] -> w428
            timing: w435 -> [_]
            timing-out: [_] -> w434
            tunnel: w424 -> [w460]
            tunnel: w423 -> [w440]
            tunnel: w422 -> [w437]
            tunnel: w420 -> [w436]
            stop <- w463 stop-if-true
            w452 = 10 ("timeout in ms (-1)")
            # "Async Read Loop"
            n150 = node-c288() -> ()  [unwired: 1 in, 1 out]
            n151 = call "Async OIM Data.vi"("error in (no error)"=w461, "Address"=w436, "Modbus Master in"=w460) -> ("error out"=w459:errorcluster, "Resistance 2"=w458:dbl, "Insulation Fault_24V"=w457:bool)  [unwired: 5 in, 1 out]
            n152 = Number To Fractional String(number=w458) -> (F-format string=w454:string)  [unwired: 3 in]
            n153 = Format Into String(format string="%s,", w457) -> (resulting string=w455:string)  [unwired: 2 in, 1 out]
            n154 = Concatenate Strings(w455, w454) -> (w439:string)
            n155 = Format Into String(format string="%s,%s", w440, w439) -> (resulting string=w438:string)  [unwired: 2 in, 1 out]
            n156 = String To Byte Array(string=w438) -> (unsigned byte array=w446:u8[])
            n157 = Array Size(array=w446) -> (size(s)=w445:i32)
            n158 = Format Date/Time String(time format string (%c)="%d:%m:%Y %H:%M:%S%.7u") -> (date/time string=w443:string)  [unwired: 2 in]
            n159 = Bundle By Name(cluster=T6 {"Command"="", "SubCmd"="", "Data"={"Port"="", "Length"=0, "Data"=[], "Time"=""}}, "Data.Time"=w443, "SubCmd"="Monitor" ("Sub Command"), "Command"="Async", "Data.Data"=w446, "Data.Length"=w445, "Data.Port"=w437) -> (w449:T6)
            n160 = Increment(x=w469) -> (x+1=w468:i32)
            n161 = Flatten To JSON(anything=w449, error in (no error)=w459) -> (JSON string=w451:string, 11:w450:errorcluster)  [unwired: 1 in]
            n162 = Enqueue Element(queue=w470, element=w451, timeout in ms (-1)=w452, error in (no error)=w450) -> (error out=w453:errorcluster)  [unwired: 2 out]
            n163 = Enqueue Element(queue=w471, element=w451, timeout in ms (-1)=w452, error in (no error)=w453) -> (error out=w467:errorcluster)  [unwired: 2 out]
            n164 = Wait on Notification(notifier=w466, timeout in ms (-1)=0, error in (no error)=w467) -> (notification=w464:bool, error out=w462:errorcluster)  [unwired: 1 in, 2 out]
            n165 = node-c288() -> ()  [unwired: 1 in, 1 out]
            n166 = Compound Arithmetic op=OR(w464, w462) -> (w463:bool)
          }
          n167 = node-c288(w434) -> ()  [unwired: 1 out]
          n168 = Merge Errors(w427, w428) -> (w429:errorcluster)
        }
      }
    }
    frame Error {
    }
  }
  "error out" <- w16
  "Device Stop" <- w9
  "Total # Send" <- w2
